vi "DtOLTimingWaveform.vi"(8 "error in (no error)":errorcluster, 10 "Waveform In":waveform(dbl)={"t0"=timestamp(0 s since 1904-01-01), "dt"=0.0, "Y"=[]}, 11 "Task in":i32) -> (0 "error out":errorcluster, 1 "Actual Freq (Hz)":dbl, 2 "Waveform Out":waveform(dbl), 3 "Task out":i32)   [LabVIEW 2022 SP3]
doc: "For analog output tasks that use the OLWaveformGenerate VI or one of LabVIEW's built-in VIs to generate waveforms, configures the timing to match the waveform."
uses:
  DtLvLink.lvlib
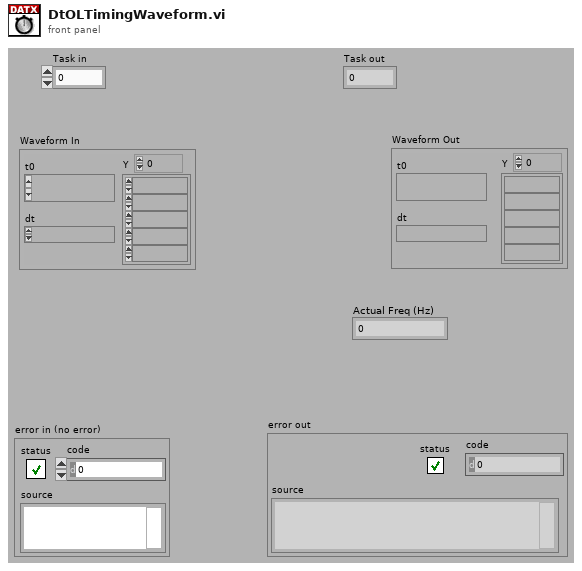
[diagram p1: front panel]
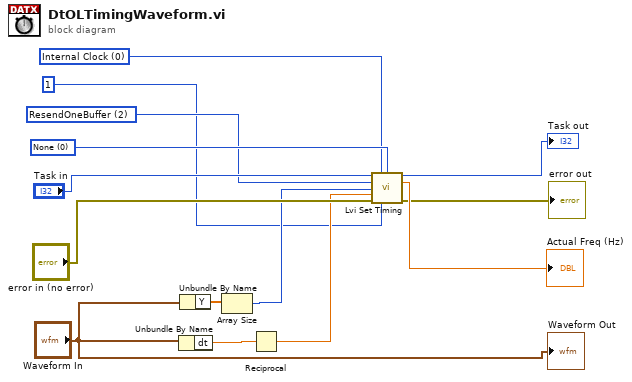
[diagram p0: block diagram]
diagram:
  w5 = 0 items=["Internal Clock", "External Clock", "Not Timed"] ("LvClockSources ClkSource")
  w6 = 0 items=["None", "Master", "Slave"] ("SynchronizationModes SyncMode")
  w4 = 2 items=["Finite", "Continuous", "ResendOneBuffer"] ("LvSampleModes SampleMode")
  n1 = Unbundle By Name("Waveform In") -> ("dt"=w9:dbl)
  n2 = Unbundle By Name("Waveform In") -> ("Y"=w8:dbl[])
  n3 = Array Size(array=w8) -> (size(s)=w3:i32)
  n4 = Reciprocal(x=w9) -> (1/x=w2:dbl)
  n5 = call "Lvi Set Timing.vi"("TaskRef"="Task in", "ClkSource"=w5, "SyncMode"=w6, "SampleMode"=w4, "PointsPerChan"=w3, "SampleRate"=w2, "error in (no error)"="error in (no error)", "NumBuffers"=u32 1 ("Int32 NumBuffers")) -> ("TaskRef out"=→"Task out":i32, "ActualSampleRate"=→"Actual Freq (Hz)":dbl, "error out"=→"error out":errorcluster)  [unwired: 4 in, 1 out]
  "Waveform Out" <- "Waveform In"
